vi "getAdditionalDataFromXMLNative.vi"(8 "error in (no error)":errorcluster, 10 "eventXML":refnum<k20>, 11 "SingleToneRamp in":refnum<class "SingleToneRamp.lvclass">) -> (0 "error out":errorcluster, 2 "eventXML out":refnum<k20>, 3 "SingleToneRamp out":refnum<class "SingleToneRamp.lvclass">)   [LabVIEW 2009, in "Tools.lvlib" / "Scripting.lvlib" / "SingleToneRamp.lvclass"]
uses:
  SingleToneRamp.lvclass
  SingleToneRamp.lvclass/SingleToneRamp.ctl
  <vilib>/xml/Close Reference(Node).vi
  <vilib>/xml/NI_XML.lvlib
  SingleTone.lvclass
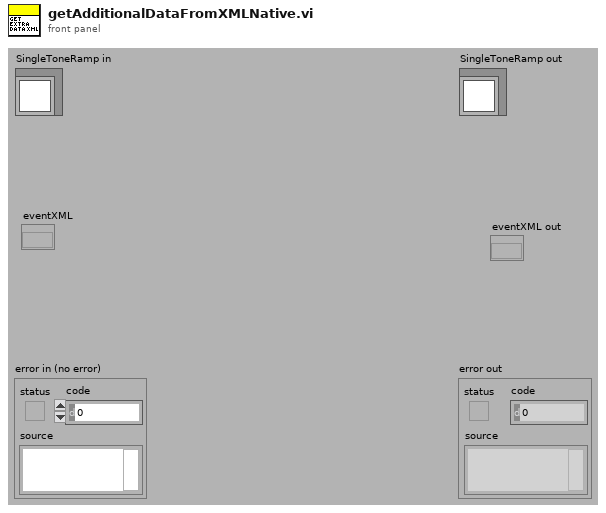
[diagram p1: front panel]
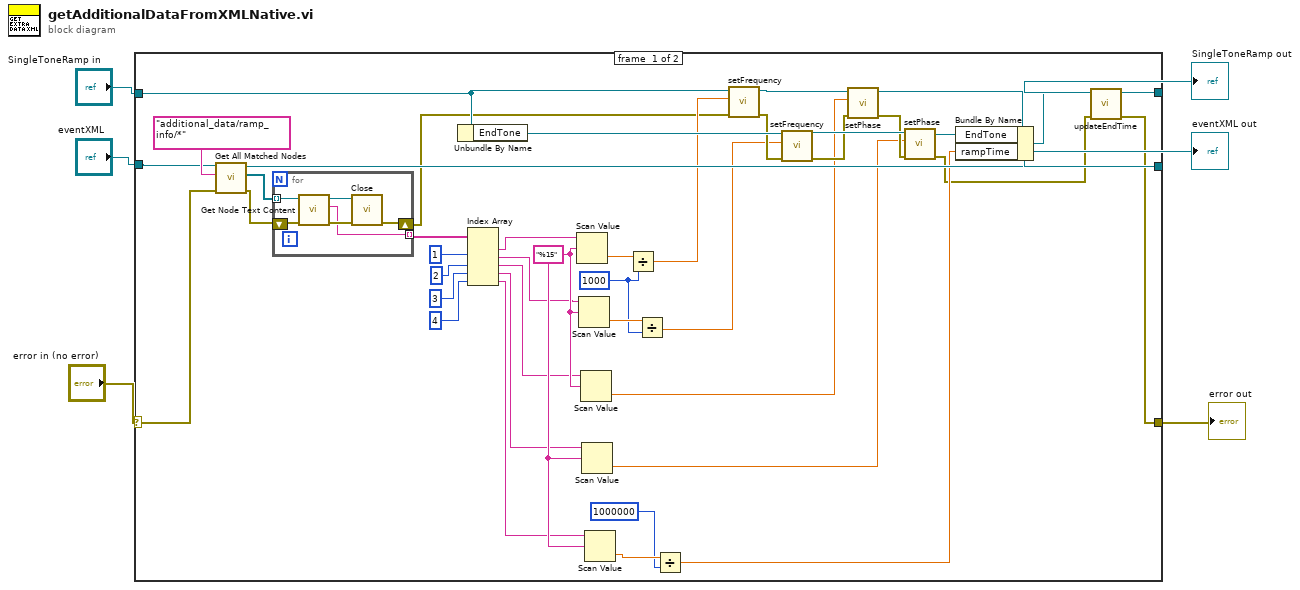
[diagram p0: block diagram]
diagram:
  n1 = case shown="No Error" "error in (no error)" {
    selector: "error in (no error)" -> [w42 w54]
    tunnel: [w7 w54] -> w1
    tunnel: "SingleToneRamp in" -> [w16 w55]
    tunnel: [w9 w55] -> w3
    tunnel: [w41 _] -> w2
    tunnel: "eventXML" -> [w40 _]
    frame #0 {
      w37 = 1000
      w36 = "%15"
      n2 = call <vilib>:"Get All Matched Nodes.vi"("error in (no error)"=w42, "XPath expression"="additional_data/ramp_info/*", "node in"=w40) -> ("error out"=w47:errorcluster, "node result array"=w45:refnum<k20>[], "node out"=w41:refnum<k20>)  [unwired: 6 in]
      n3 = for {
        tunnel: w45 -> [w50] mode=indexing
        tunnel: [w49] -> w44 mode=indexing
        shift-right: [w48] -> w14
        shift-left: w47 -> [w51]
        n4 = call <vilib>:"Get Node Text Content.vi"("error in (no error)"=w51, "node in"=w50) -> ("error out"=w52:errorcluster, "node text"=w49:string, "node out"=w53:refnum<k20>)  [unwired: 7 in]
        n5 = call-poly <vilib>:"Close.vi"("error in (no error)"=w52, "node"=w53) -> ("error out"=w48:errorcluster)  [unwired: 7 in]
      }
      n6 = Unbundle By Name(w16) -> ("EndTone"=w25:refnum<class "SingleTone.lvclass">)
      n7 = Index Array(array=w44, index #2=1 ("index"), index #3=2 ("index"), index #4=3 ("index"), index #5=4 ("index")) -> (element #1=w30:string, element #2=w29:string, element #3=w28:string, element #4=w27:string, element #5=w26:string)  [unwired: 1 in]
      n8 = Scan Value(string=w30, format string=w36) -> (value=w39:dbl)  [unwired: 1 in, 1 out]
      n9 = Scan Value(string=w29, format string=w36) -> (value=w38:dbl)  [unwired: 1 in, 1 out]
      n10 = Scan Value(string=w28, format string=w36) -> (value=w12:dbl)  [unwired: 1 in, 1 out]
      n11 = Scan Value(string=w27, format string=w36) -> (value=w11:dbl)  [unwired: 1 in, 1 out]
      n12 = Scan Value(string=w26, format string=w36) -> (value=w35:dbl)  [unwired: 1 in, 1 out]
      n13 = Divide(x=w39, y=w37) -> (x/y=w15:dbl)
      n14 = Divide(x=w38, y=w37) -> (x/y=w13:dbl)
      n15 = Divide(x=w35, y=1000000) -> (x/y=w10:dbl)
      n16 = call "setFrequency.vi"("error in (no error)"=w14, "frequency"=w15, "SingleTone.lvclass in"=w16) -> ("error out"=w24:errorcluster, "SingleTone.lvclass out"=w23:refnum<class "SingleToneRamp.lvclass">)  [unwired: 7 in]
      n17 = call "setFrequency.vi"("error in (no error)"=w24, "frequency"=w13, "SingleTone.lvclass in"=w25) -> ("error out"=w21:errorcluster, "SingleTone.lvclass out"=w22:refnum<class "SingleTone.lvclass">)  [unwired: 7 in]
      n18 = call "setPhase.vi"("error in (no error)"=w21, "phase"=w12, "SingleTone.lvclass in"=w23) -> ("error out"=w20:errorcluster, "SingleTone.lvclass out"=w19:refnum<class "SingleToneRamp.lvclass">)  [unwired: 7 in]
      n19 = call "setPhase.vi"("error in (no error)"=w20, "phase"=w11, "SingleTone.lvclass in"=w22) -> ("error out"=w8:errorcluster, "SingleTone.lvclass out"=w18:refnum<class "SingleTone.lvclass">)  [unwired: 7 in]
      n20 = Bundle By Name(cluster=w19, "EndTone"=w18, "rampTime"=w10) -> (w17:refnum<class "SingleToneRamp.lvclass">)
      n21 = call-dynamic "updateEndTime.vi"("error in (no error)"=w8, "SingleToneRamp in"=w17) -> ("error out"=w7:errorcluster, "SingleToneRamp out"=w9:refnum<class "SingleToneRamp.lvclass">)  [unwired: 8 in]
    }
    frame #1 {
    }
  }
  "error out" <- w1
  "SingleToneRamp out" <- w3
  "eventXML out" <- w2
